vi "ConvertToStandJSON.vi"(8 "error in (no error)":errorcluster, 11 "caps":string) -> (0 "error out":errorcluster, 3 "json caps":string)   [LabVIEW 2017, in "Paser.lvlib"]
uses:
  Paser.lvlib
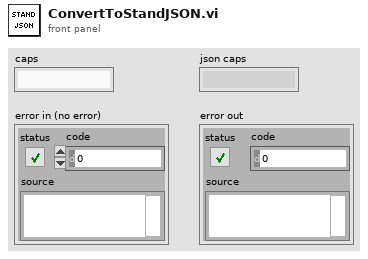
[diagram p1: front panel]
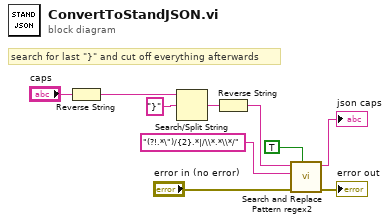
[diagram p0: block diagram]
diagram:
  # "search for last \"}\" and cut off everything afterwards"
  n1 = Reverse String(1:"caps") -> (0:w3:string)
  n2 = Search/Split String(string=w3, search string/char (-)="}") -> (match + rest of string=w6:string)  [unwired: 1 in, 2 out]
  n3 = Reverse String(1:w6) -> (0:w5:string)
  n4 = call "Search and Replace Pattern regex2.vi"("replace all? (F)"=TRUE, "error in"="error in (no error)", "regular expression (\"\")"="(?!.*\")/{2}.*|/\\*.*\\*/" ("regular expression (\"\")"), "string"=w5) -> ("error out"=→"error out":errorcluster, "result string"=→"json caps":string)  [unwired: 5 in, 1 out]
